vi "niFpga_LRMGlobalCount.vi"() -> ()   [LabVIEW 2017]
panel:
  in  "Count":u32
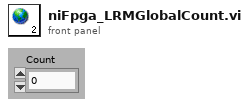
[diagram p1: front panel]
diagram:
